vi "Plot Descr Write.vi"(4 "error in (no error)":errorcluster, 5 "Value":T1(array[cluster]), 6 "Container State":T3, 7 "Display State In":T2) -> (0 "error out":errorcluster, 3 "Display State Out":T2)   [LabVIEW 2013, in "1D Buffer.xctl"]
uses:
  1D Buffer.xctl
  <vilib>/_xctls/Container State.ctl
  State.ctl
  <vilib>/_xctls/XControlSupport.lvlib
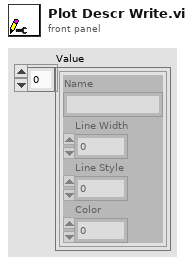
[diagram p1: front panel]
types:
  T1 = cluster{"Name":string, "Line Width":u8, "Line Style":u8, "Color":u32}[]
  T2 = typedef "1D Buffer.xctl/State.ctl" = cluster{"Data Array":sgl[][], "Time Array":timestamp[], "History":u16, "Variable":bool[], "Plot Details":cluster{"Name":string, "Line Width":u8, "Line Style":u8, "Color":u32}[], "Y-Axis Labels":string[], "legend visible":bool}
  T3 = typedef "XControlSupport.lvlib/Container State.ctl" = cluster{"Indicator?":bool, "Run Mode?":bool, " Refnum":refnum<vi>}
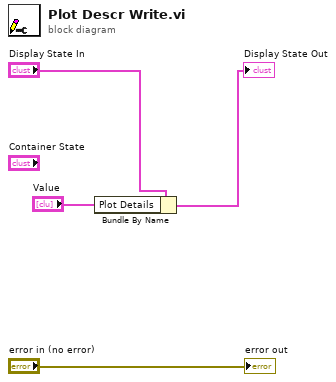
[diagram p0: block diagram]
diagram:
  n1 = Bundle By Name(cluster="Display State In", "Plot Details"="Value") -> (→"Display State Out":T2)
  "error out" <- "error in (no error)"
